vi "Menu-Stop Acq EOC.vi"(11 "Menu in":refnum<k9>) -> ()   [LabVIEW 2019, in "CML UI.lvlib"]
uses:
  CML UI.lvlib
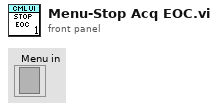
[diagram p1: front panel]
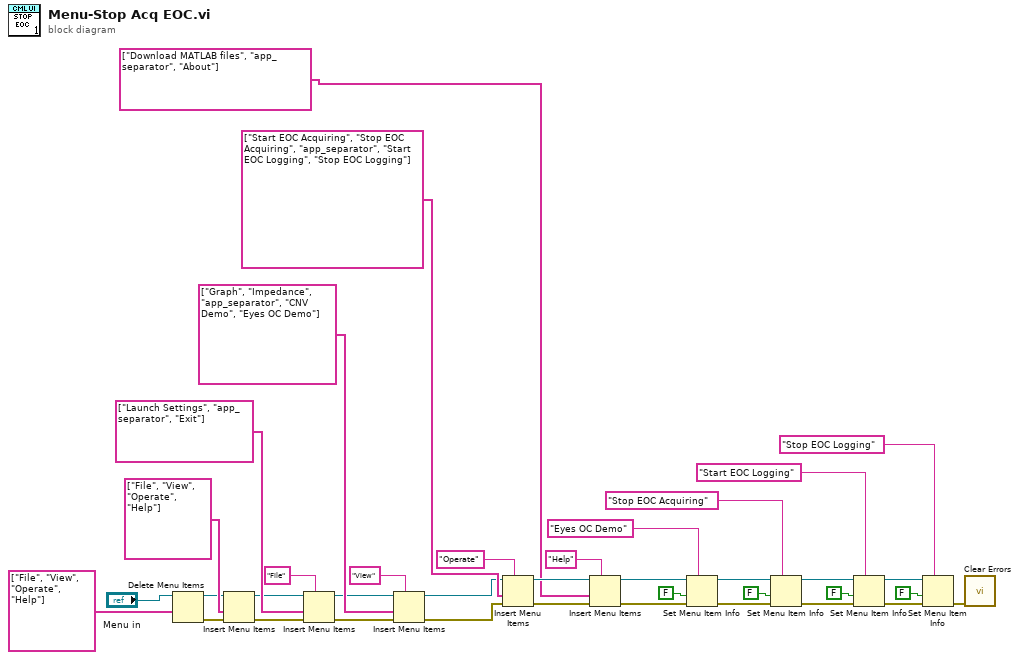
[diagram p0: block diagram]
diagram:
  n1 = Delete Menu Items(7:string[] ["File", "View", "Operate", "Help"] ("L10n_item tags 1"), 9:"Menu in") -> (0:w14:errorcluster, 3:w15:refnum<k9>)  [unwired: 2 in]
  n2 = Insert Menu Items(6:w14, 7:string[] ["File", "View", "Operate", "Help"] ("L10n_item tags 1"), 9:w15) -> (0:w27:errorcluster, 3:w25:refnum<k9>)  [unwired: 3 in, 1 out]
  n3 = Insert Menu Items(5:"File" ("L10n_menu tag"), 6:w27, 7:string[] ["Launch Settings", "app_separator", "Exit"] ("L10n_item tags 2"), 9:w25) -> (0:w32:errorcluster, 3:w31:refnum<k9>)  [unwired: 2 in, 1 out]
  n4 = Insert Menu Items(5:"View" ("L10n_menu tag"), 6:w32, 7:string[] ["Graph", "Impedance", "app_separator", "CNV Demo", "Eyes OC Demo"] ("L10n_item tags 2"), 9:w31) -> (0:w36:errorcluster, 3:w35:refnum<k9>)  [unwired: 2 in, 1 out]
  n5 = Insert Menu Items(5:"Operate" ("L10n_menu tag"), 6:w36, 7:string[] ["Start EOC Acquiring", "Stop EOC Acquiring", "app_separator", "Start EOC Logging", "Stop EOC Logging"] ("L10n_item tags 2"), 9:w35) -> (0:w22:errorcluster, 3:w23:refnum<k9>)  [unwired: 2 in, 1 out]
  n6 = Insert Menu Items(5:"Help" ("L10n_menu tag"), 6:w22, 7:string[] ["Download MATLAB files", "app_separator", "About"] ("L10n_item tags 2"), 9:w23) -> (0:w19:errorcluster, 3:w21:refnum<k9>)  [unwired: 2 in, 1 out]
  n7 = Set Menu Item Info(7:"Eyes OC Demo" ("item tag"), 8:w19, 9:FALSE ("enabled"), 11:w21) -> (0:w8:errorcluster, 3:w9:refnum<k9>)  [unwired: 3 in]
  n8 = Set Menu Item Info(7:"Stop EOC Acquiring" ("item tag"), 8:w8, 9:FALSE ("enabled"), 11:w9) -> (0:w6:errorcluster, 3:w7:refnum<k9>)  [unwired: 3 in]
  n9 = Set Menu Item Info(7:"Start EOC Logging" ("item tag"), 8:w6, 9:FALSE ("enabled"), 11:w7) -> (0:w4:errorcluster, 3:w5:refnum<k9>)  [unwired: 3 in]
  n10 = Set Menu Item Info(7:"Stop EOC Logging" ("item tag"), 8:w4, 9:FALSE ("enabled"), 11:w5) -> (0:w2:errorcluster)  [unwired: 3 in, 1 out]
  n11 = call <vilib>:"Clear Errors.vi"("error in (no error)"=w2) -> ()  [unwired: 5 in, 2 out]
